vi "Advection_Velocity.vi"() -> (0 "New Values In":string[][](array[string])=[["Test data5"]], 1 "New Chs In":string[](array[string])=["30-10-03:New:Channel new5"])   [LabVIEW 2021]
uses:
  Data plotting/subVIs/Plot_Values_Global.vi
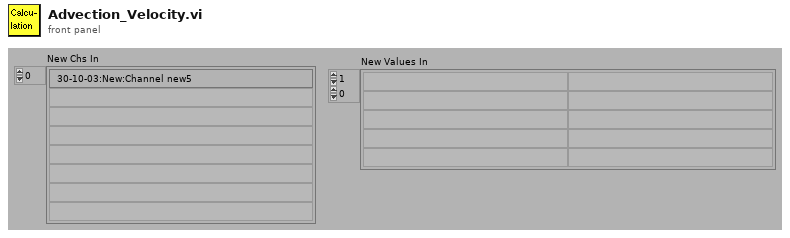
[diagram p1: front panel]
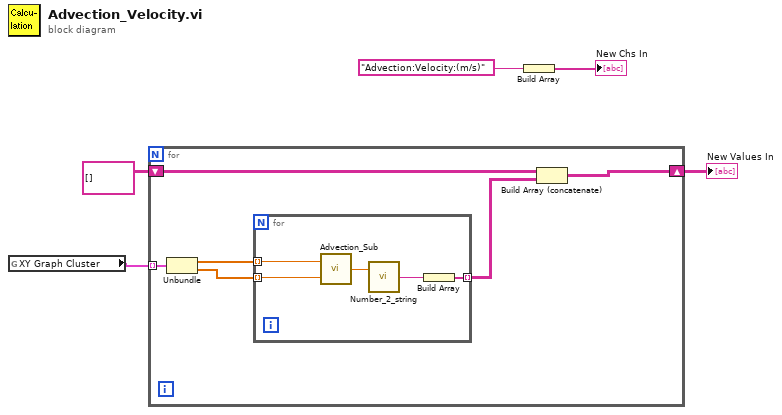
[diagram p0: block diagram]
diagram:
  n1 = global read "Plot_Values_Global.vi" "XY Graph Cluster"() -> (w1:cluster{dbl[], dbl[]}[])
  n2 = for {
    tunnel: w1 -> [w11] mode=indexing
    shift-right: [w9] -> w3
    shift-left: string[][] [] -> [w10]
    n3 = Unbundle(w11) -> (w8:dbl[], w7:dbl[])
    n4 = for {
      tunnel: w8 -> [w16] mode=indexing
      tunnel: w7 -> [w15] mode=indexing
      tunnel: [w12] -> w6 mode=indexing
      n5 = call "Advection_Sub.vi"("Uref"=w15, "Z"=w16) -> ("U m/s"=w14:dbl)
      n6 = call "Number_2_string.vi"("number"=w14) -> ("String"=w13:string)  [unwired: 1 in]
      n7 = Build Array(w13) -> (w12:string[])
    }
    n8 = Build Array (concatenate)(w10, w6) -> (w9:string[][])
  }
  "New Values In" <- w3
  n9 = Build Array("Advection:Velocity:(m/s)" ("string")) -> (→"New Chs In":string[])
